vi "斯坦道溶解氧校准.vi"() -> ()   [LabVIEW 2016, in "斯坦道多参数.lvlib"]
uses:
  <vilib>/Utility/miscctls.llb/LVPointTypeDef.ctl
  <vilib>/Analysis/NI_AALBase.lvlib
  <vilib>/Analysis/NI_AALPro.lvlib
panel:
  in  "读取":bool
  out "滤波设定":dbl
  out "第二点信号值":dbl
  out "第一点信号值":dbl
  out "通讯状态":string
  in  "盐度自动获取":bool
  in  "大气压补偿":dbl format="%#.2f"
  in  "盐度补偿":dbl format="%#.2f"
  out "DO %":dbl caption="饱和度值" format="%#.2f"
  out "第二点校准值":dbl
  out "第一点校准值":dbl
  out "最小值":sgl format="%.2g"
  out "最大值":sgl format="%.2g"
  in  "校准停止":bool
  in  "校准模式":u16(ring) items=["两点校准", "单点校准"]
  in  "标液2":dbl
  in  "标液1":dbl
  out "波形图表":dbl(graph) caption="历史曲线"
  out "温度测量值":dbl caption="温度" format="%#.2f"
  out "变异系数":dbl format="%.6g"
  out "standard deviation":dbl caption="标准差" format="%0.2f"
  out "mean":dbl caption="均值" format="%0.2f"
  out "提示":string
  in  "校准启动":bool
  out "DO mg/L":dbl caption="测试值" format="%#.2f"
  out "电极斜率":dbl format="%#.6f"
  out "电极零点":dbl format="%#.6f"
  # "溶解氧电极设定"
  # "℃"
  # "%"
  # "mg/L"
  # "kPa"
  # "请选择校准模式:"
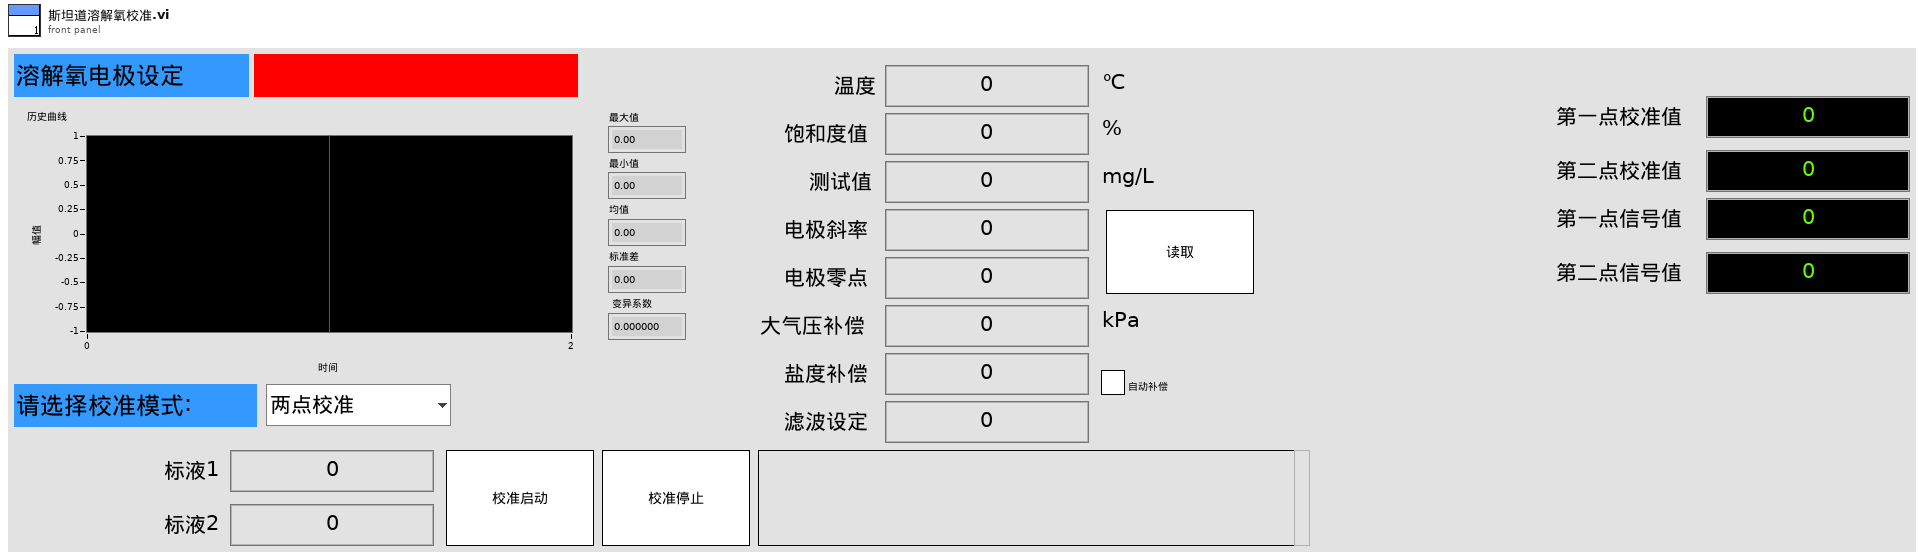
[diagram p1: front panel]
types:
  T1 = typedef "斯坦道多参数.lvlib/通知队列类型.ctl" = enum16{"pH", "DO", "DO2", "Cond", "Turb", "ORP", "叶绿素a", "藻密度", "COD"}
  T2 = typedef "LVPointTypeDef.ctl" = cluster{"Horizontal":i16, "Vertical":i16}
  T3 = cluster{"pH":u32, "DO":u32, "Cond":u32, "Turb":u32, "叶绿素a":u32, "藻密度":u32, "ORP":u32, "COD":u32}
  T4 = enum8{"Enabled", "Disabled", "Disabled and Grayed Out"}
  T5 = cluster{"ph":bool, "DO":bool, "Cond":bool, "Turb":bool, "叶绿素a":bool, "藻密度":bool, "ORP":bool, "COD":bool, "DO2":bool}
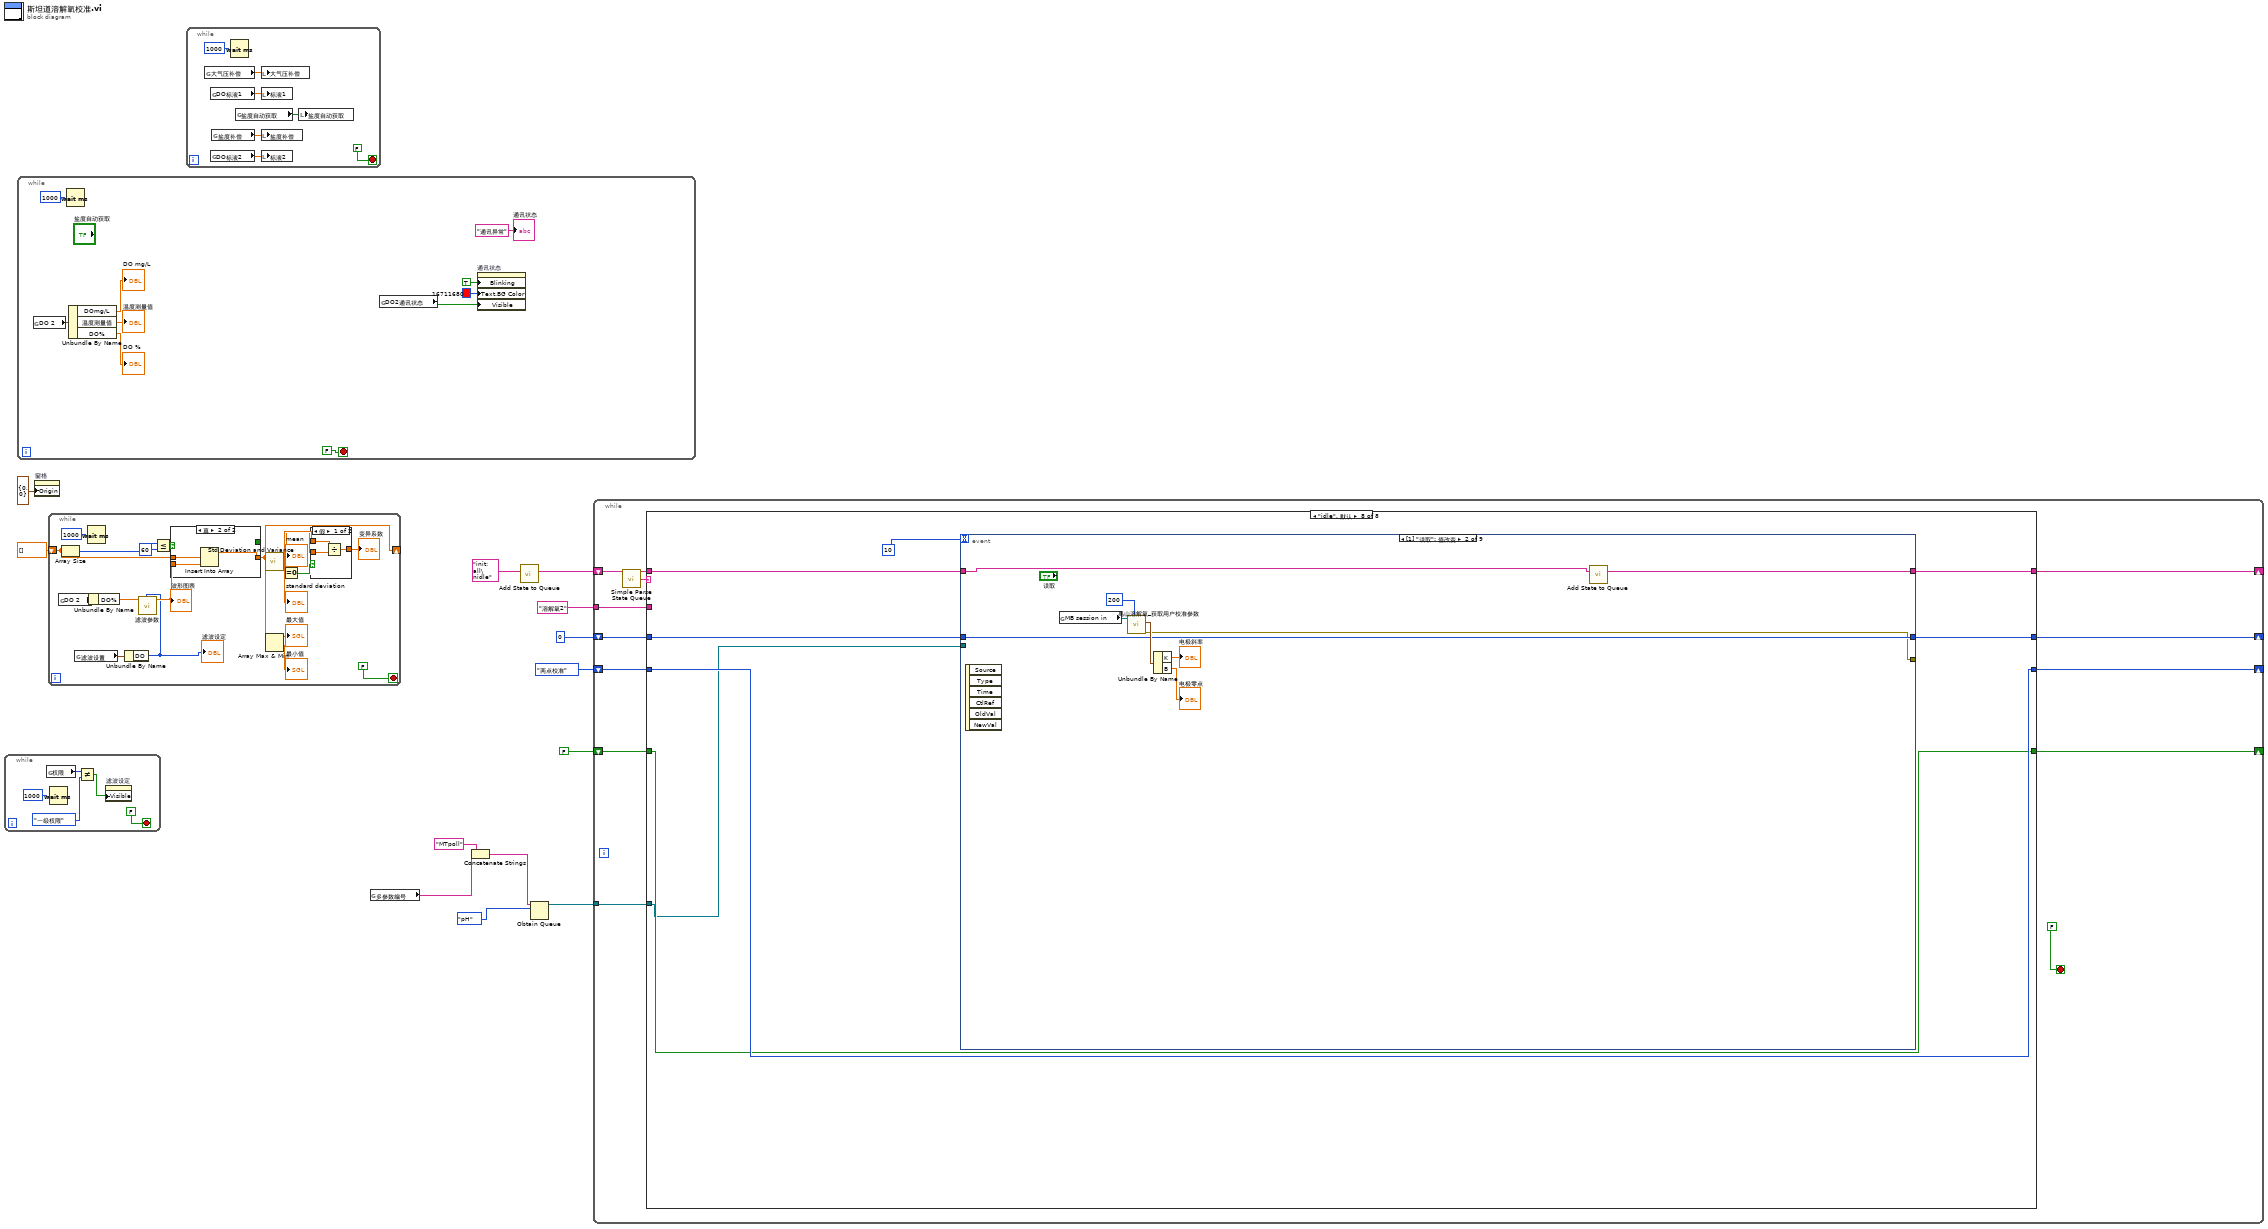
[diagram p0: block diagram]
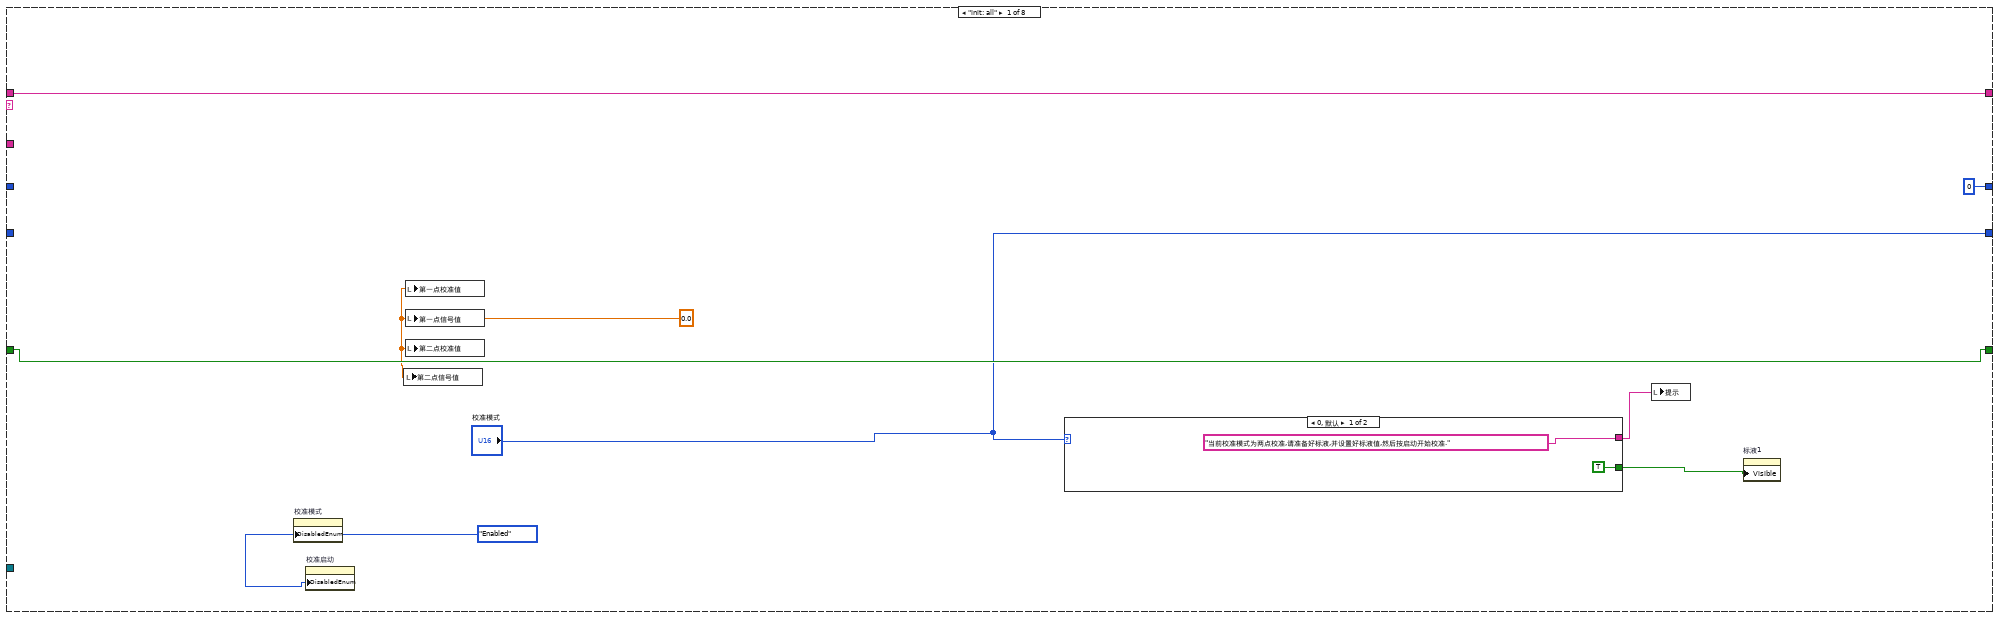
[diagram p2: hidden frame]
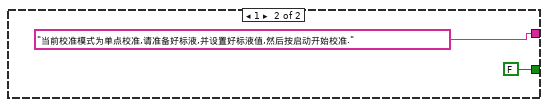
[diagram p3: hidden frame]
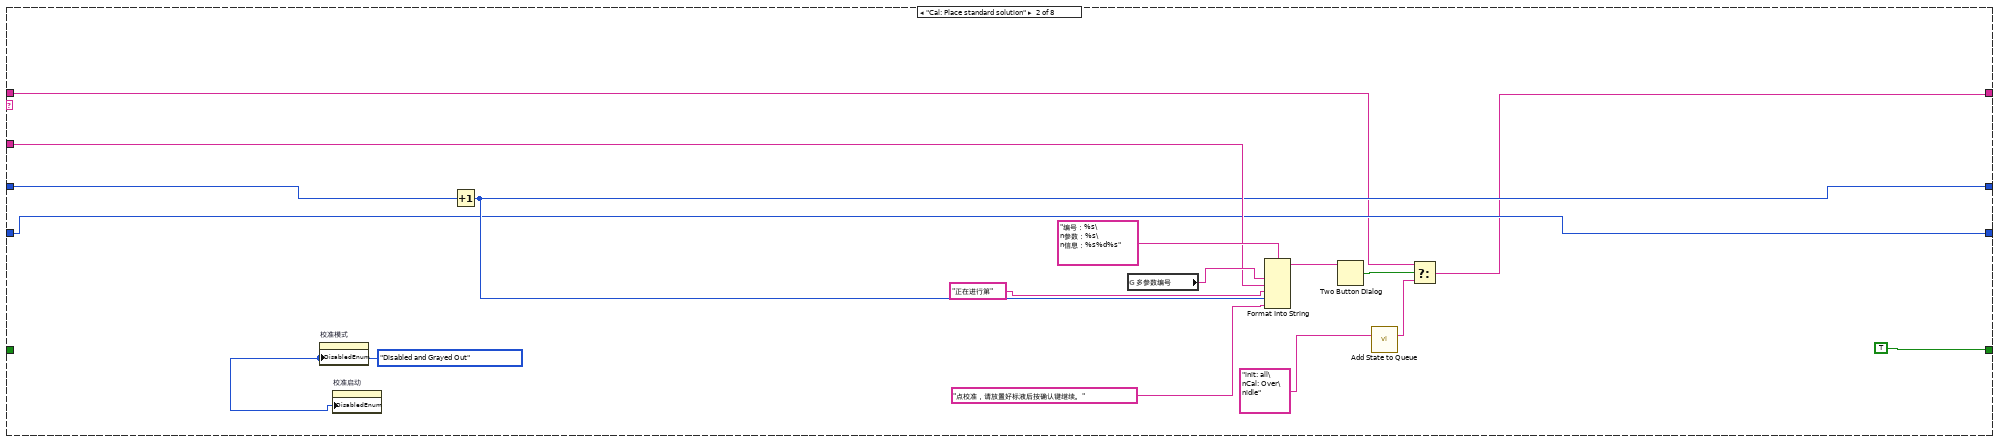
[diagram p4: hidden frame]
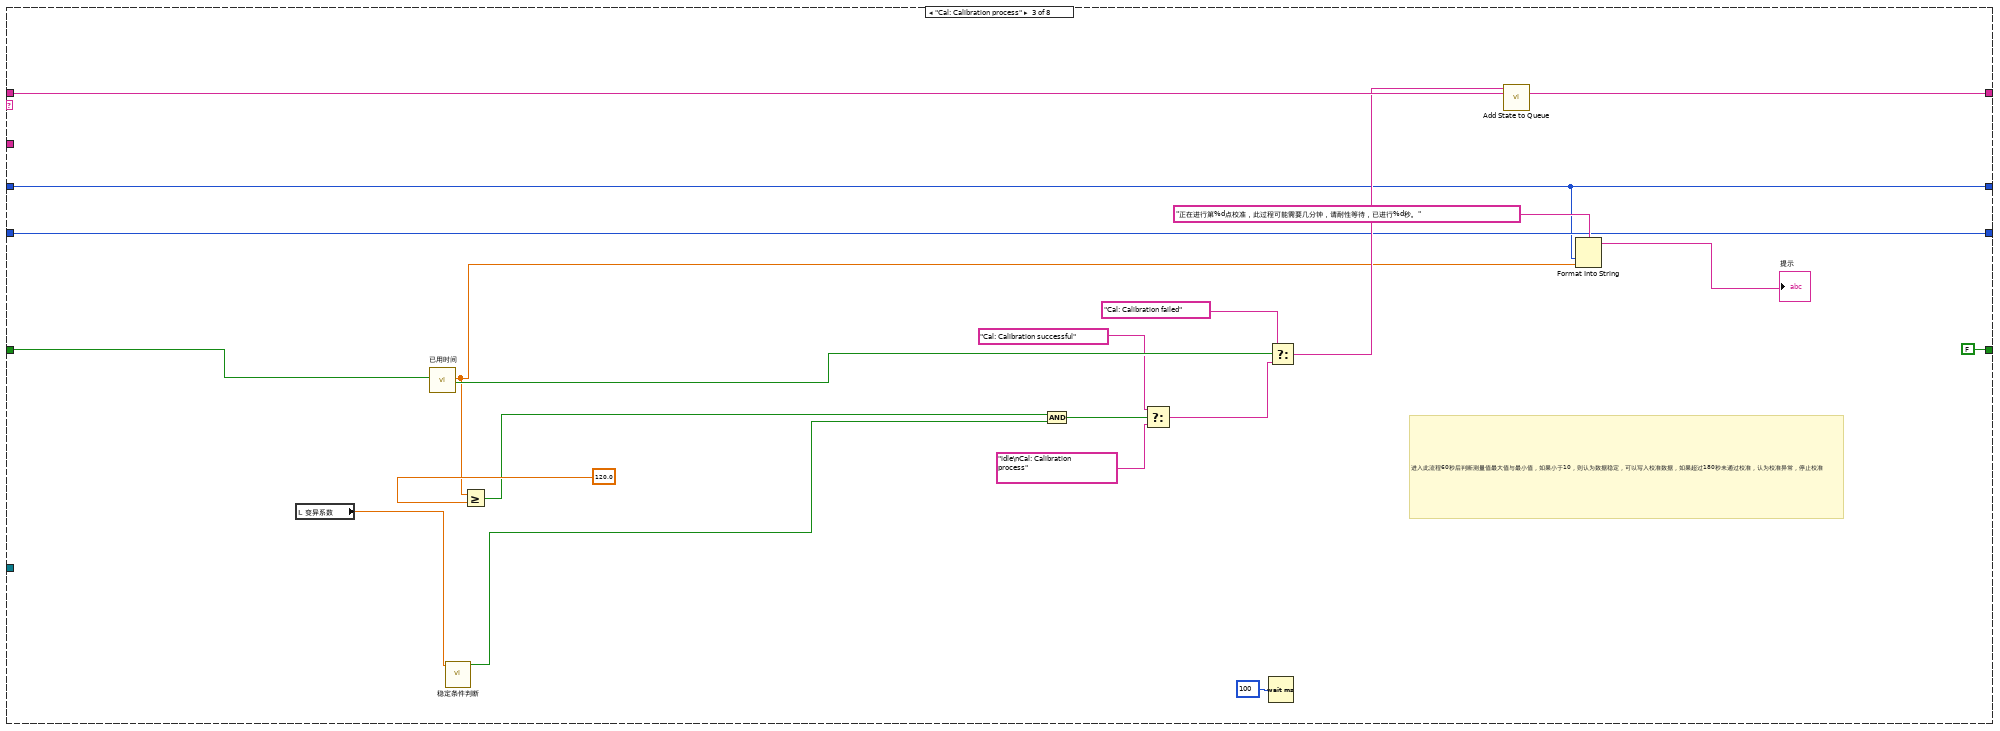
[diagram p5: hidden frame]
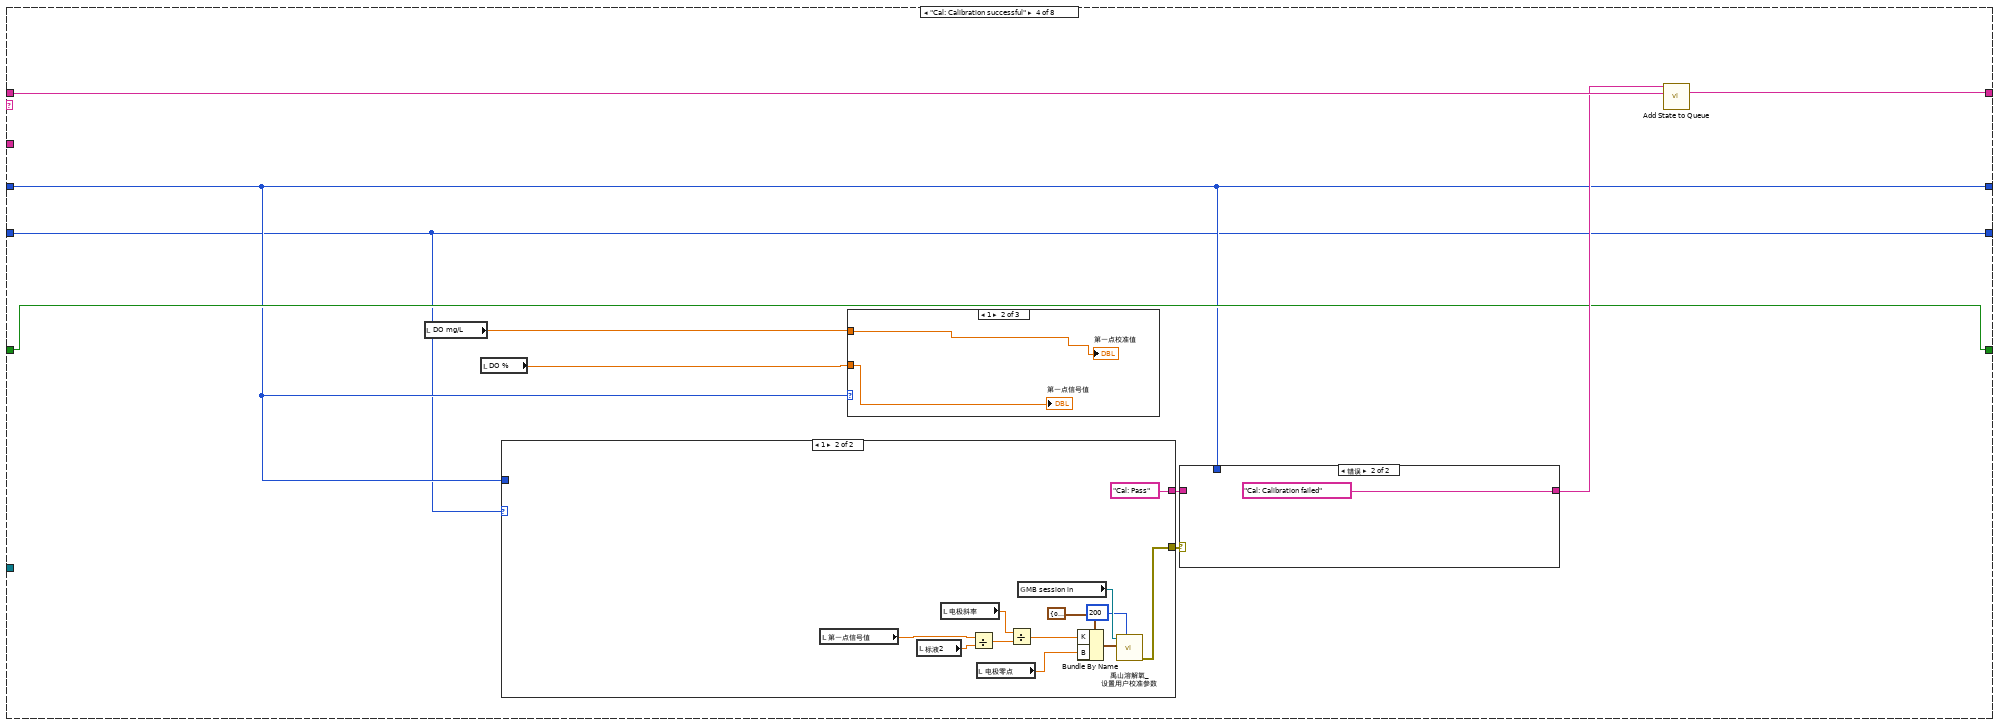
[diagram p6: hidden frame]
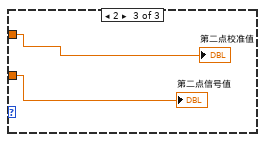
[diagram p8: hidden frame]
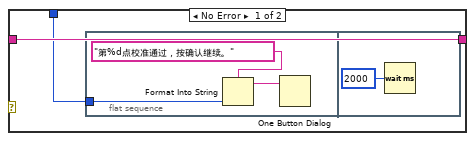
[diagram p9: hidden frame]
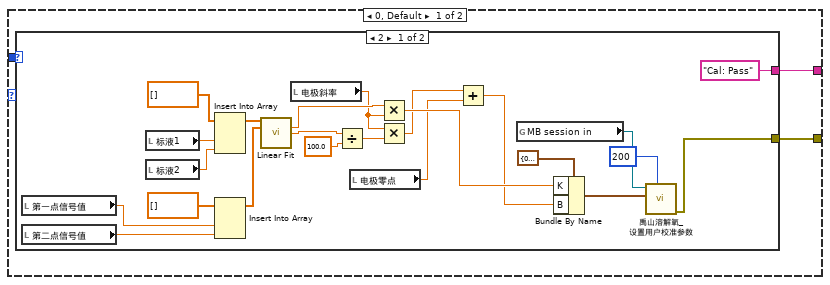
[diagram p10: hidden frame]
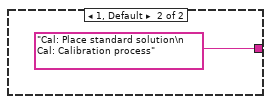
[diagram p11: hidden frame]
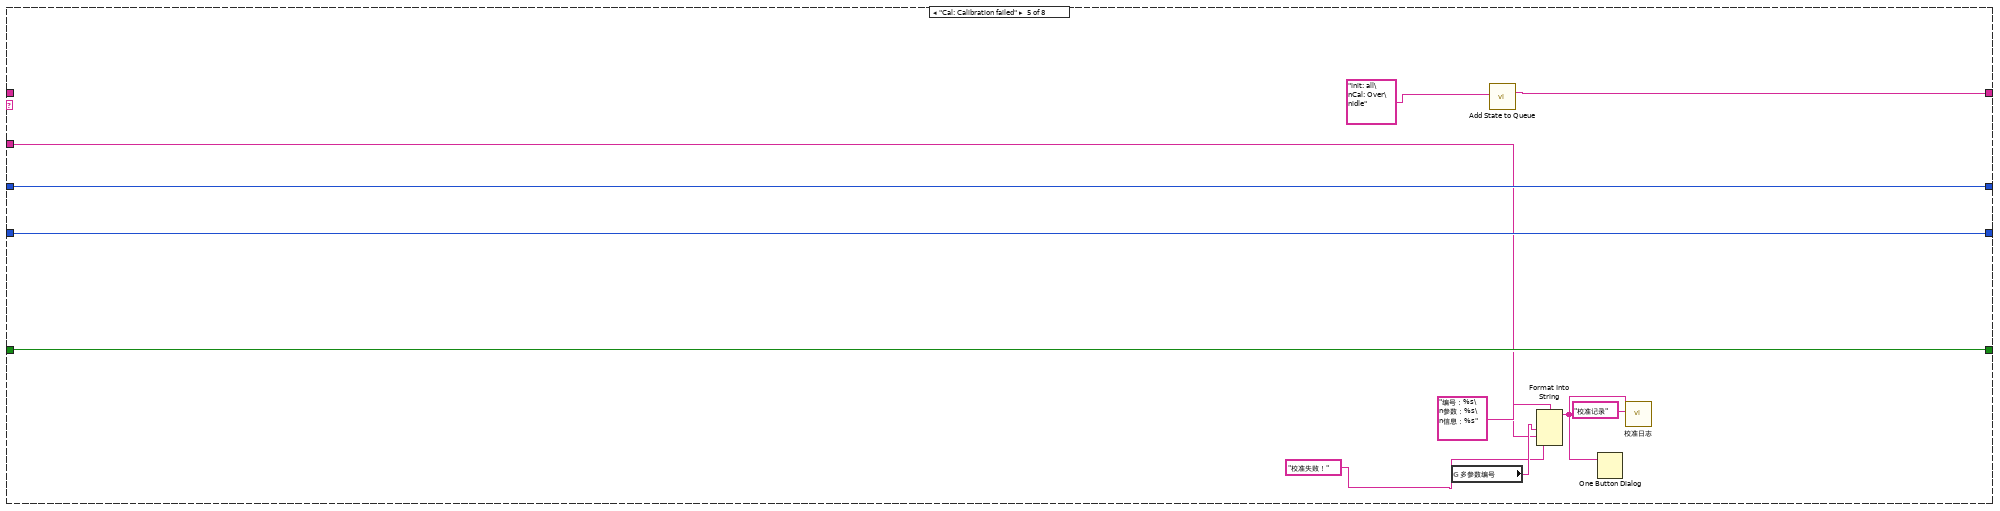
[diagram p12: hidden frame]
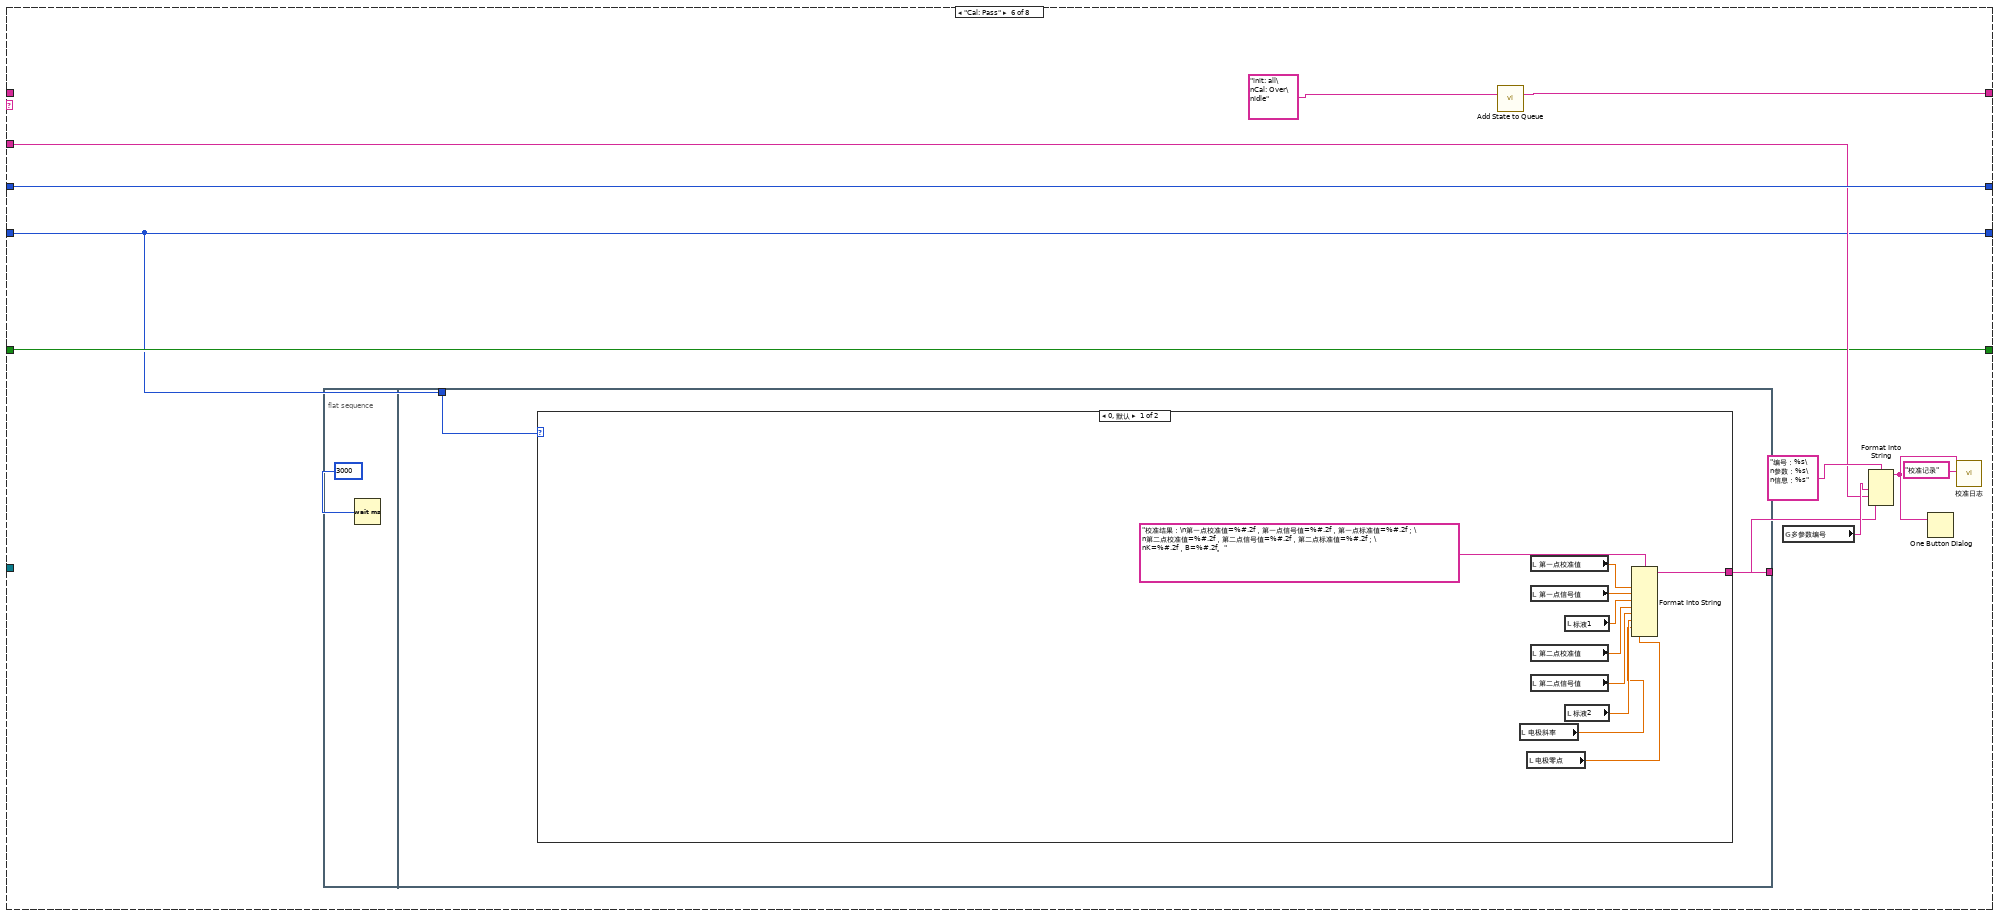
[diagram p13: hidden frame]
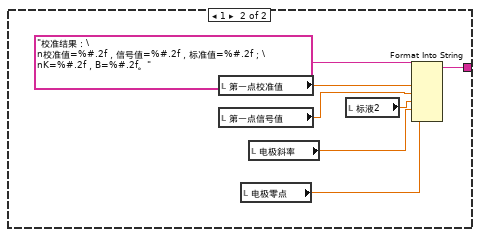
[diagram p14: hidden frame]
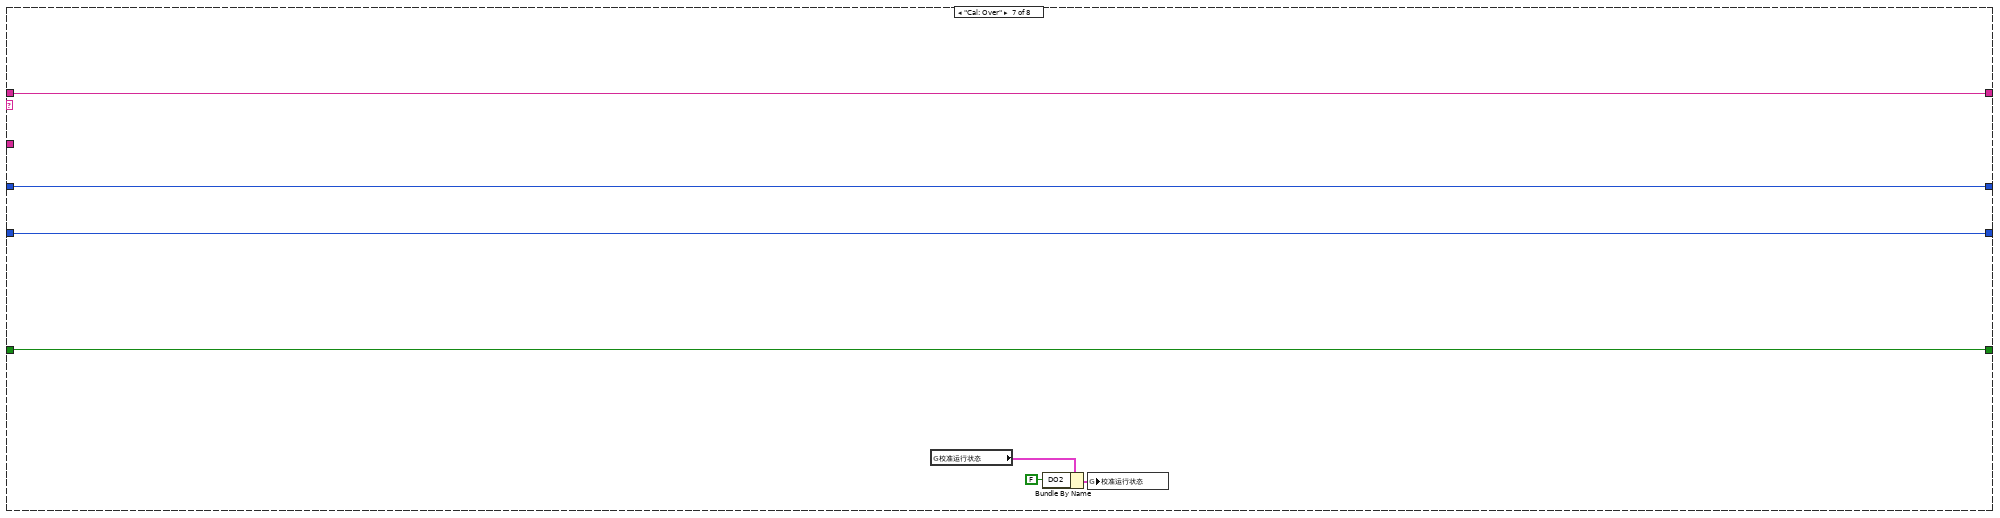
[diagram p15: hidden frame]
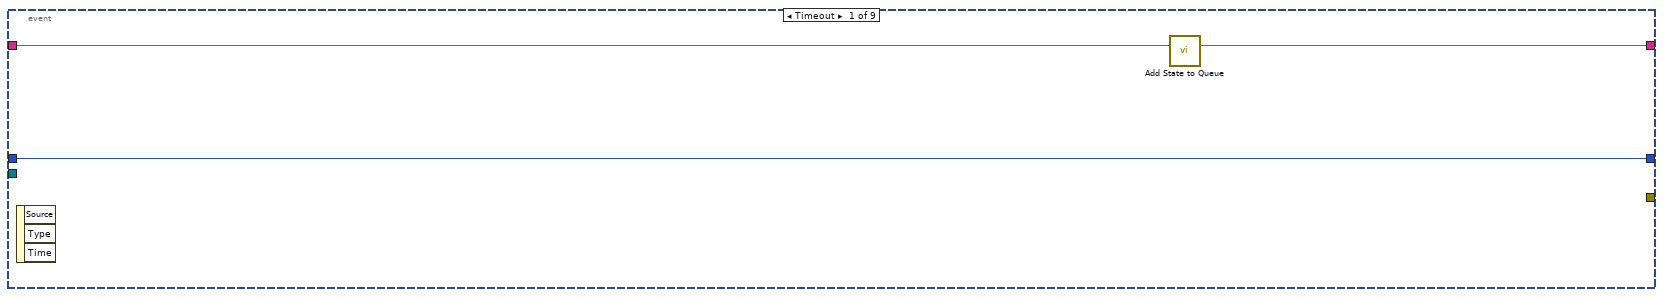
[diagram p16: hidden frame]
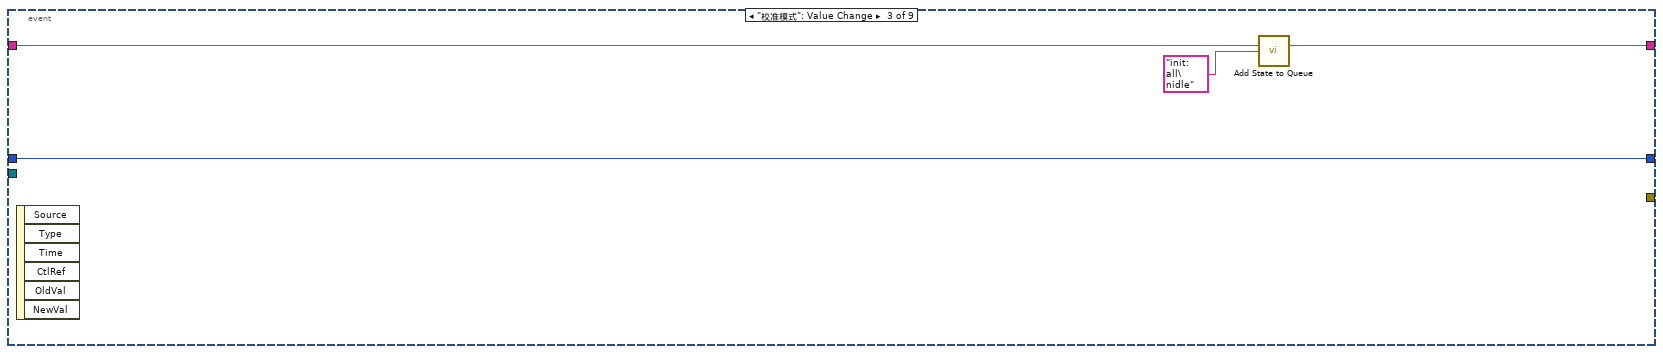
[diagram p17: hidden frame]
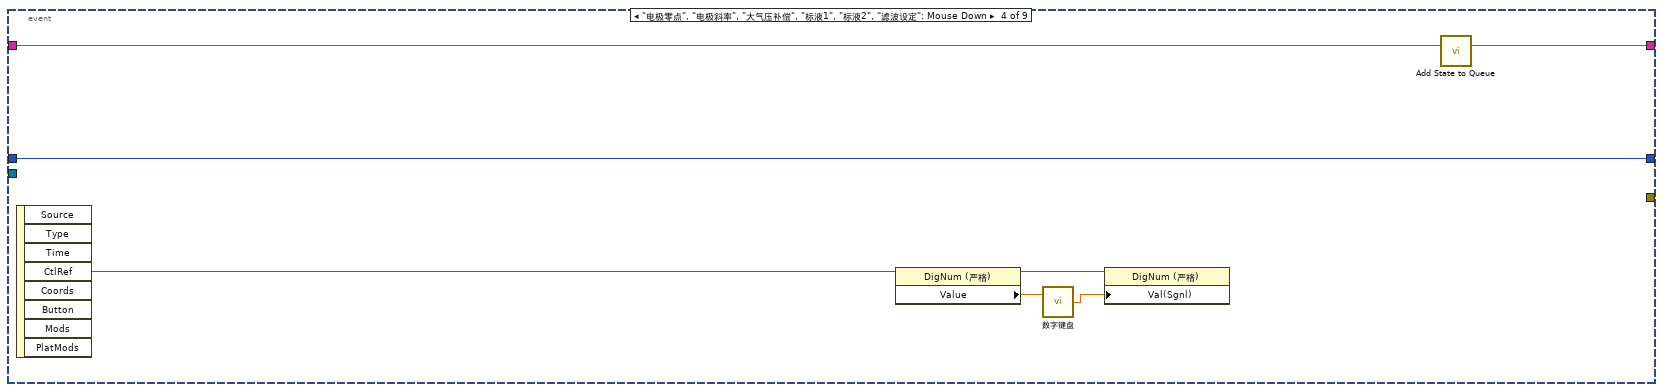
[diagram p18: hidden frame]
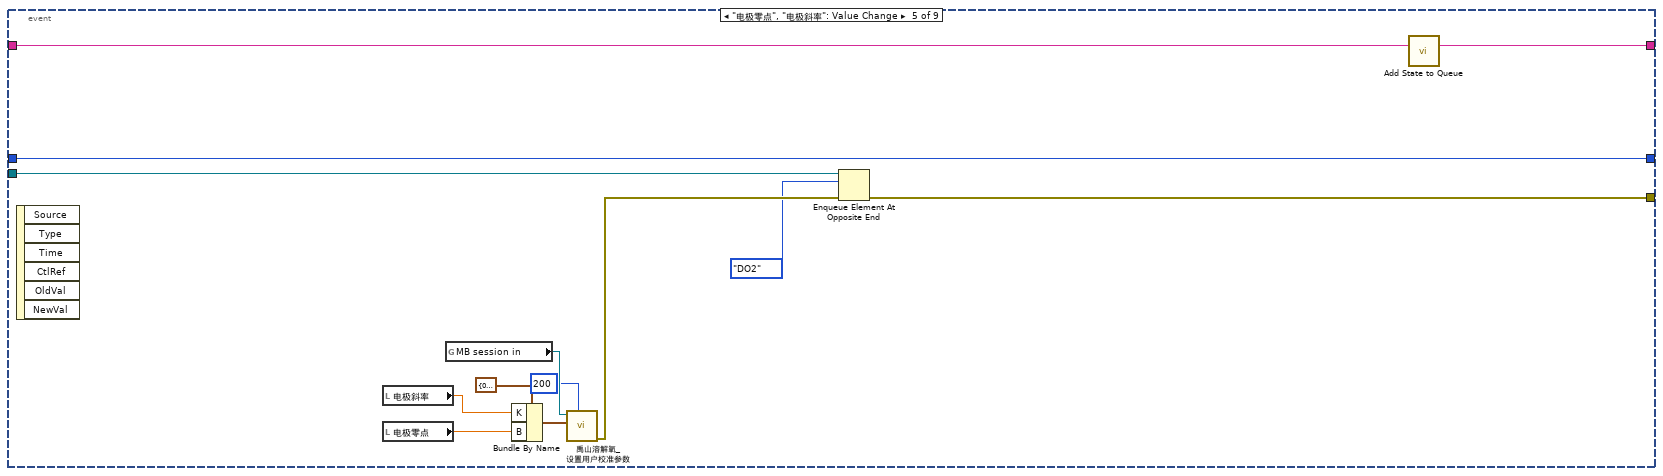
[diagram p19: hidden frame]
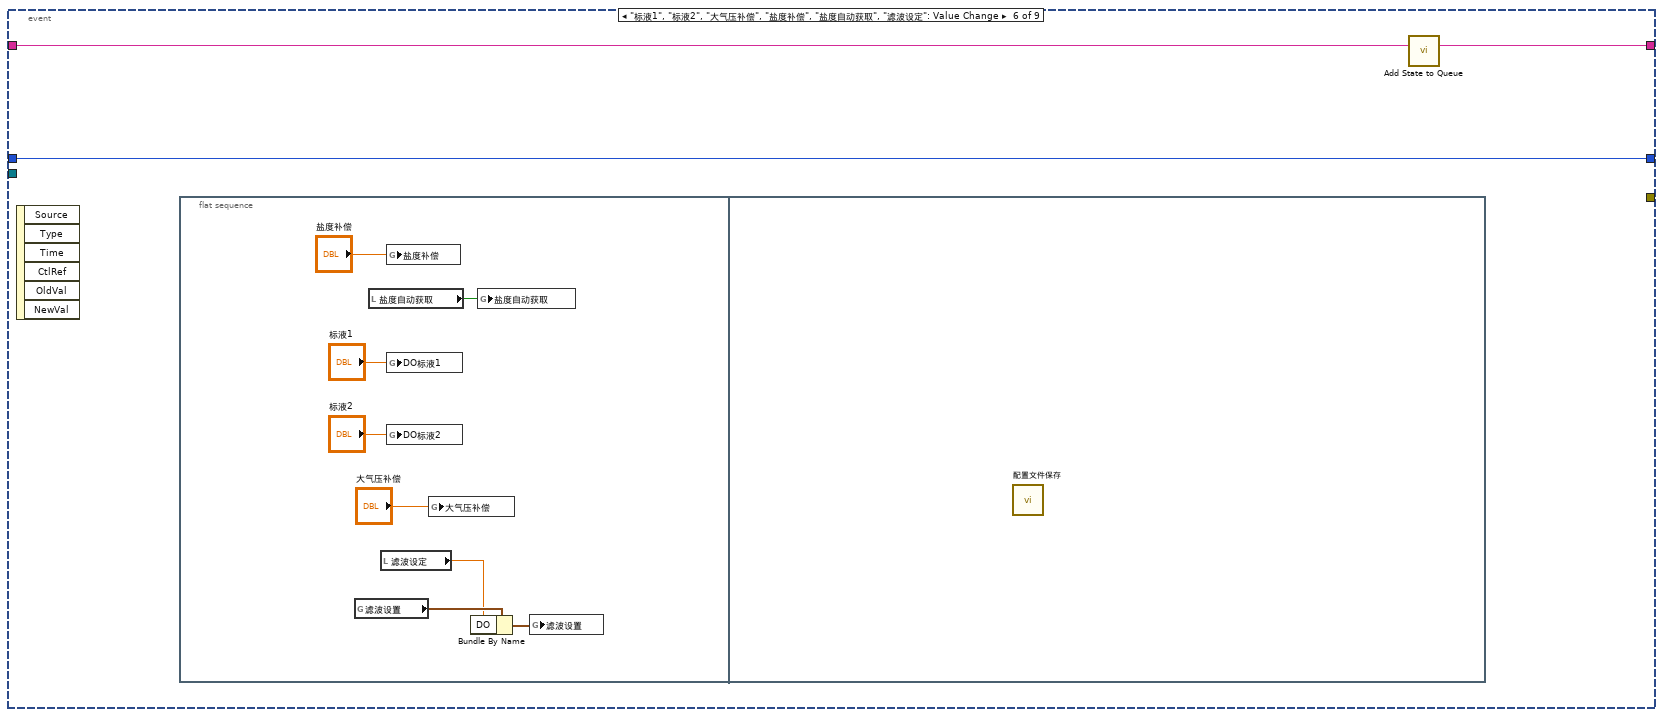
[diagram p20: hidden frame]
diagram:
  n1 = while {
    stop <- FALSE stop-if-true
    n2 = global read "多参数全局变量.vi" "权限"() -> (w17:enum16{"一级权限", "二级权限", "三级权限"})
    n3 = Wait (ms)(milliseconds to wait=u32 1000 ("等待时间（毫秒）")) -> ()  [unwired: 1 out]
    n4 = Not Equal?(x=w17, y=enum16{"一级权限", "二级权限", "三级权限"}."一级权限") -> (x != y?=w14:bool)
    n5 = property on="滤波设定" class="DigNum (严格)"("Visible"=w14) -> ()  [unwired: 2 in, 2 out]
  }
  n6 = while {
    stop <- FALSE stop-if-true
    n7 = global read "禹山过程全局变量.vi" "DO 2"() -> (w24:cluster{"温度测量值":sgl, "DO%":sgl, "DOmg/L":sgl})
    n8 = Wait (ms)(milliseconds to wait=u32 1000 ("等待时间（毫秒）")) -> ()  [unwired: 1 out]
    n9 = Unbundle By Name(w24) -> ("DOmg/L"=→"DO mg/L":sgl, "温度测量值"=→"温度测量值":sgl, "DO%"=→"DO %":sgl)
    n10 = global read "多参数全局变量.vi" "DO2通讯状态"() -> (w19:bool)
    n11 = property on="通讯状态" class="Str"("Blinking"=TRUE ("闪烁"), "Text.BG Color"=u32 16711680, "Visible"=w19) -> ()  [unwired: 2 in, 2 out]
    "通讯状态" <- "通讯异常" ("当前串口")
  }
  n12 = property on="窗格" class="Pane"("Origin"=T2 {"Horizontal"=0, "Vertical"=0} ("原点")) -> ()  [unwired: 2 in, 2 out]
  n13 = while {
    shift-right: [w35] -> _
    shift-left: sgl[] [] -> [w42]
    stop <- FALSE stop-if-true
    n14 = global read "禹山过程全局变量.vi" "DO 2"() -> (w36:cluster{"温度测量值":sgl, "DO%":sgl, "DOmg/L":sgl})
    n15 = Array Size(array=w42) -> (size(s)=w44:i32)
    n16 = global read "断电保存变量.vi" "滤波设置"() -> (w30:T3)
    n17 = Wait (ms)(milliseconds to wait=u32 1000 ("等待时间（毫秒）")) -> ()  [unwired: 1 out]
    n18 = Unbundle By Name(w36) -> ("DO%"=w32:sgl)
    n19 = Unbundle By Name(w30) -> ("DO"=w29:u32)
    "滤波设定" <- w29
    n20 = call "滤波参数.vi"("滤波次数"=w29, "x"=w32) -> ("mode"=w31:dbl)  [unwired: 9 in]
    "波形图表" <- w31
    n21 = Less Or Equal?(x=w44, y=60) -> (x <= y?=w43:bool)
    n22 = case shown="真" w43 {
      tunnel: w42 -> [w55 w58]
      tunnel: w31 -> [w53 w57]
      tunnel: [w51 w56] -> w35
      tunnel: [TRUE _] -> _
      frame False {
        n23 = Replace Array Subset(array=w55, new element=w53) -> (w54:sgl[])  [unwired: 1 in]
        n24 = Rotate 1D Array(1:w54, 2:-1 ("n")) -> (0:w51:sgl[])
      }
      frame True {
        n25 = Insert Into Array(array=w58, new element=w57) -> (w56:sgl[])  [unwired: 1 in]
      }
    }
    n26 = call <vilib>:"Std Deviation and Variance.vi"("X"=w35) -> ("mean"=w37:dbl, "standard deviation"=w38:dbl)  [unwired: 1 in, 1 out]
    "standard deviation" <- w38
    "mean" <- w37
    n27 = Array Max & Min(array=w35) -> (max value=→"最大值":sgl, min value=→"最小值":sgl)  [unwired: 2 out]
    n28 = Equal To 0?(x=w37) -> (x = 0?=w41:bool)
    n29 = case shown="假" w41 {
      tunnel: w38 -> [w49 _]
      tunnel: [w48 _] -> w40
      tunnel: w37 -> [w47 _]
      frame False {
        n30 = Divide(x=w49, y=w47) -> (x/y=w48:dbl)
      }
      frame True {
      }
    }
    "变异系数" <- w40
  }
  n31 = while {
    stop <- FALSE stop-if-true
    n32 = global read "断电保存变量.vi" "大气压补偿"() -> (w61:dbl)
    n33 = global read "断电保存变量.vi" "DO标液1"() -> (w63:dbl)
    n34 = global read "断电保存变量.vi" "DO标液2"() -> (w62:dbl)
    n35 = global read "断电保存变量.vi" "盐度补偿"() -> (w59:dbl)
    n36 = Wait (ms)(milliseconds to wait=u32 1000 ("等待时间（毫秒）")) -> ()  [unwired: 1 out]
    n37 = global read "断电保存变量.vi" "盐度自动获取"() -> (w60:bool)
    n38 = local write "大气压补偿"(w61) -> ()
    n39 = local write "标液1"(w63) -> ()
    n40 = local write "盐度补偿"(w59) -> ()
    n41 = local write "标液2"(w62) -> ()
    n42 = local write "盐度自动获取"(w60) -> ()
  }
  n43 = global read "多参数全局变量.vi" "多参数编号"() -> (w3:string)
  n44 = Concatenate Strings("MTpoll" ("名称（未命名）"), w3) -> (w4:string)
  n45 = call "Add State to Queue.vi"("State(s) In (\"\")"="init: all\nidle" ("State(s) In (\"\")")) -> ("States Out"=w10:string)  [unwired: 14 in]
  n46 = Obtain Queue(name (unnamed)=w4, element data type=通知队列类型."pH" ("枚举")) -> (queue out=w2:refnum<queue>)  [unwired: 3 in, 2 out]
  n47 = while {
    shift-right: [w74] -> _
    shift-left: w10 -> [w78]
    shift-right: [w71] -> _
    shift-left: 0 -> [w73]
    tunnel: "溶解氧2" ("State(s) In (\"\")") -> [w72]
    shift-right: [w69] -> _
    shift-left: enum16{"两点校准", "单点校准"}."两点校准" ("校准模式") -> [w70]
    shift-right: [w67] -> _
    shift-left: FALSE -> [w68]
    tunnel: w2 -> [w66]
    stop <- FALSE stop-if-true
    n48 = call "Simple Parse State Queue.vi"("State Queue"=w78) -> ("Remain States"=w75:string, "Next State"=w76:string)  [unwired: 13 in]
    n49 = case shown="\"idle\", 默认" w76 {
      tunnel: w75 -> [w86 w94 w126 w135 _ _ w236 w244]
      tunnel: [w86 w93 w125 w134 w195 w200 w236 w243] -> w74
      tunnel: w73 -> [_ w102 w111 w129 w198 w209 w235 w241]
      tunnel: w72 -> [_ w103 _ _ w189 w205 _ _]
      tunnel: [0 w100 w111 w129 w198 w209 w235 w242] -> w71
      tunnel: w70 -> [_ w99 w112 w128 w197 w201 w234 w240]
      tunnel: ["校准模式" w99 w112 w128 w197 w201 w234 w240] -> w69
      tunnel: w68 -> [w83 _ w114 w130 w196 w204 w233 w238]
      tunnel: [w83 TRUE FALSE w130 w196 w204 w233 w238] -> w67
      tunnel: w66 -> [_ _ _ _ _ _ _ w237]
      frame "init: all" {
        w81 = T4."Enabled" ("禁用")
        w82 = 0.0 ("第一点校准值")
        n50 = property on="校准模式" class="Ring (严格)"("DisabledEnum"=w81) -> ()  [unwired: 2 in, 2 out]
        n51 = property on="校准启动" class="Bool"("DisabledEnum"=w81) -> ()  [unwired: 2 in, 2 out]
        n52 = local write "第二点信号值"(w82) -> ()
        n53 = local write "第一点校准值"(w82) -> ()
        n54 = local write "第一点信号值"(w82) -> ()
        n55 = local write "第二点校准值"(w82) -> ()
        n56 = case shown="0, 默认" "校准模式" {
          tunnel: ["当前校准模式为两点校准,请准备好标液,并设置好标液值,然后按启动开始校准." ("提示") "当前校准模式为单点校准,请准备好标液,并设置好标液值,然后按启动开始校准." ("提示")] -> w85
          tunnel: [TRUE ("可见") FALSE ("可见")] -> w79
          frame 0, Default {
          }
          frame 1 {
          }
        }
        n57 = local write "提示"(w85) -> ()
        n58 = property on="标液1" class="DigNum (严格)"("Visible"=w79) -> ()  [unwired: 2 in, 2 out]
      }
      frame "Cal: Place standard solution" {
        w92 = T4."Disabled and Grayed Out" ("禁用")
        n59 = property on="校准模式" class="Ring (严格)"("DisabledEnum"=w92) -> ()  [unwired: 2 in, 2 out]
        n60 = property on="校准启动" class="Bool"("DisabledEnum"=w92) -> ()  [unwired: 2 in, 2 out]
        n61 = Increment(x=w102) -> (x+1=w100:i32)
        n62 = global read "多参数全局变量.vi" "多参数编号"() -> (w105:string)
        n63 = Format Into String(format string="编号：%s\n参数：%s\n信息：%s%d%s" ("格式字符串"), w105, w103, "正在进行第" ("消息"), w100, "点校准，请放置好标液后按确认键继续。" ("消息")) -> (resulting string=w97:string)  [unwired: 2 in, 1 out]
        n64 = Two Button Dialog(message=w97) -> (T button?=w96:bool)  [unwired: 2 in]
        n65 = call "Add State to Queue.vi"("State(s) In (\"\")"="init: all\nCal: Over\nidle" ("State(s) In (\"\")")) -> ("States Out"=w95:string)  [unwired: 14 in]
        n66 = Select(t=w94, s=w96, f=w95) -> (s? t:f=w93:string)
      }
      frame "Cal: Calibration process" {
        # "进入此流程60秒后判断测量值最大值与最小值，如果小于10，则认为数据稳定，可以写入校准数据，如果超过180秒未通过校准，认为校准异常，停止校准"
        n67 = local read "变异系数"() -> (w108:dbl)
        n68 = call "已用时间"("Reset"=w114) -> ("Elapsed Time (s)"=w110:dbl, "Time has Elapsed"=w127:bool)  [unwired: 11 in, 6 out]
        n69 = call "稳定条件判断.vi"("变异系数"=w108) -> ("布尔"=w107:bool)  [unwired: 10 in]
        n70 = Greater Or Equal?(x=w110, y=120.0) -> (x >= y?=w122:bool)
        n71 = And(x=w122, y=w107) -> (x .and. y?=w119:bool)
        n72 = Select(t="Cal: Calibration successful" ("State(s) In (\"\")"), s=w119, f="idle\nCal: Calibration process" ("State(s) In (\"\")")) -> (s? t:f=w118:string)
        n73 = Wait (ms)(milliseconds to wait=u32 100 ("等待时间（毫秒）")) -> ()  [unwired: 1 out]
        n74 = Select(t="Cal: Calibration failed" ("State(s) In (\"\")"), s=w127, f=w118) -> (s? t:f=w117:string)
        n75 = call "Add State to Queue.vi"("State(s) In Front (\"\")"=w117, "State(s) In (\"\")"=w126) -> ("States Out"=w125:string)  [unwired: 13 in]
        n76 = Format Into String(format string="正在进行第%d点校准，此过程可能需要几分钟，请耐性等待，已进行%d秒。" ("格式字符串"), w111, w110) -> (resulting string=→"提示":string)  [unwired: 2 in, 1 out]
      }
      frame "Cal: Calibration successful" {
        n77 = local read "DO mg/L"() -> (w131:dbl)
        n78 = local read "DO %"() -> (w132:dbl)
        n79 = case shown="1" w128 {
          tunnel: [w151 w177] -> w137
          tunnel: [w150 "Cal: Pass" ("State(s) In (\"\")")] -> w136
          tunnel: w129 -> [w149 _]
          frame 0, Default {
            n80 = case shown="2" w149 {
              tunnel: [w153 _] -> w151
              tunnel: ["Cal: Pass" ("State(s) In (\"\")") "Cal: Place standard solution\n Cal: Calibration process" ("State(s) In (\"\")")] -> w150
              frame 2 {
                n81 = local read "第一点信号值"() -> (w172:dbl)
                n82 = local read "第二点信号值"() -> (w171:dbl)
                n83 = local read "标液1"() -> (w169:dbl)
                n84 = local read "标液2"() -> (w168:dbl)
                n85 = Insert Into Array(array=dbl[] [] ("Weight"), new element #1=w169, new element #2=w168) -> (w167:dbl[])  [unwired: 1 in]
                n86 = Insert Into Array(array=dbl[] [] ("Weight"), new element #1=w172, new element #2=w171) -> (w166:dbl[])  [unwired: 1 in]
                n87 = call <vilib>:"Linear Fit.vi"("Y"=w167, "X"=w166) -> ("slope"=w162:dbl, "intercept"=w159:dbl)  [unwired: 9 in, 3 out]
                n88 = local read "电极斜率"() -> (w160:dbl)
                n89 = Divide(x=w159, y=100.0) -> (x/y=w155:dbl)
                n90 = local read "电极零点"() -> (w157:dbl)
                n91 = Multiply(x=w162, y=w160) -> (x*y=w161:dbl)
                n92 = Multiply(x=w160, y=w155) -> (x*y=w158:dbl)
                n93 = Add(x=w158, y=w157) -> (x+y=w156:dbl)
                n94 = global read "多参数全局变量.vi" "MB session in"() -> (w165:refnum<class "MB_Master.lvclass">)
                n95 = Bundle By Name(cluster=cluster{"K":sgl, "B":sgl} {"K"=0.0, "B"=0.0} ("用户校准参数"), "K"=w161, "B"=w156) -> (w164:cluster{"K":sgl, "B":sgl})
                n96 = call "禹山溶解氧_设置用户校准参数.vi"("Slave ID"=u8 200, "用户校准参数"=w164, "MB session in"=w165) -> ("error out"=w153:errorcluster)  [unwired: 7 in, 1 out]
              }
              frame 1, Default {
              }
            }
          }
          frame 1 {
            n97 = local read "第一点信号值"() -> (w182:dbl)
            n98 = local read "标液2"() -> (w181:dbl)
            n99 = local read "电极斜率"() -> (w179:dbl)
            n100 = Divide(x=w182, y=w181) -> (x/y=w178:dbl)
            n101 = local read "电极零点"() -> (w183:dbl)
            n102 = Divide(x=w179, y=w178) -> (x/y=w180:dbl)
            n103 = global read "多参数全局变量.vi" "MB session in"() -> (w186:refnum<class "MB_Master.lvclass">)
            n104 = Bundle By Name(cluster=cluster{"K":sgl, "B":sgl} {"K"=0.0, "B"=0.0} ("用户校准参数"), "K"=w180, "B"=w183) -> (w185:cluster{"K":sgl, "B":sgl})
            n105 = call "禹山溶解氧_设置用户校准参数.vi"("Slave ID"=u8 200, "用户校准参数"=w185, "MB session in"=w186) -> ("error out"=w177:errorcluster)  [unwired: 7 in, 1 out]
          }
        }
        n106 = case shown="1" w129 {
          tunnel: w132 -> [_ w139 w141]
          tunnel: w131 -> [_ w138 w140]
          frame 0, Default {
          }
          frame 1 {
            "第一点信号值" <- w139
            "第一点校准值" <- w138
          }
          frame 2 {
            "第二点信号值" <- w141
            "第二点校准值" <- w140
          }
        }
        n107 = case shown="错误" w137 {
          tunnel: w136 -> [w143 _]
          tunnel: [w143 "Cal: Calibration failed" ("State(s) In (\"\")")] -> w133
          tunnel: w129 -> [w142 _]
          frame No Error {
            n108 = flat-sequence {
              tunnel: w142 -> [w144]
              frame #0 {
                n109 = Format Into String(format string="第%d点校准通过，按确认继续。" ("格式字符串"), w144) -> (resulting string=w146:string)  [unwired: 2 in, 1 out]
                n110 = One Button Dialog(message=w146) -> ()  [unwired: 1 in, 1 out]
              }
              frame #1 {
                n111 = Wait (ms)(milliseconds to wait=u32 2000 ("等待时间（毫秒）")) -> ()  [unwired: 1 out]
              }
            }
          }
          frame Error {
          }
        }
        n112 = call "Add State to Queue.vi"("State(s) In Front (\"\")"=w133, "State(s) In (\"\")"=w135) -> ("States Out"=w134:string)  [unwired: 13 in]
      }
      frame "Cal: Calibration failed" {
        n113 = global read "多参数全局变量.vi" "多参数编号"() -> (w192:string)
        n114 = call "Add State to Queue.vi"("State(s) In (\"\")"="init: all\nCal: Over\nidle" ("State(s) In (\"\")")) -> ("States Out"=w195:string)  [unwired: 14 in]
        n115 = Format Into String(format string="编号：%s\n参数：%s\n信息：%s" ("格式字符串"), w192, w189, "校准失败！" ("消息")) -> (resulting string=w191:string)  [unwired: 2 in, 1 out]
        n116 = One Button Dialog(message=w191) -> ()  [unwired: 1 in, 1 out]
        n117 = call "校准日志.vi"("table"="校准记录", "日志信息"=w191) -> ()  [unwired: 9 in, 1 out]
      }
      frame "Cal: Pass" {
        n118 = flat-sequence {
          tunnel: [w212] -> w202
          tunnel: w201 -> [w211]
          frame #0 {
            n119 = Wait (ms)(milliseconds to wait=u32 3000 ("等待时间（毫秒）")) -> ()  [unwired: 1 out]
          }
          frame #1 {
            n120 = case shown="0, 默认" w211 {
              tunnel: [w222 w229] -> w212
              frame 0, Default {
                n121 = local read "电极斜率"() -> (w214:dbl)
                n122 = local read "电极零点"() -> (w213:dbl)
                n123 = local read "第一点校准值"() -> (w220:dbl)
                n124 = local read "第一点信号值"() -> (w221:dbl)
                n125 = local read "第二点校准值"() -> (w217:dbl)
                n126 = local read "第二点信号值"() -> (w216:dbl)
                n127 = local read "标液1"() -> (w218:dbl)
                n128 = local read "标液2"() -> (w215:dbl)
                n129 = Format Into String(format string="校准结果：\n第一点校准值=%#.2f，第一点信号值=%#.2f，第一点标准值=%#.2f；\n第二点校准值=%#.2f，第二点信号值=%#.2f，第二点标准值=%#.2f；\nK=%#.2f，B=%#.2f。" ("提示"), w220, w221, w218, w217, w216, w215, w214, w213) -> (resulting string=w222:string)  [unwired: 2 in, 1 out]
              }
              frame 1 {
                n130 = local read "第一点校准值"() -> (w228:dbl)
                n131 = local read "第一点信号值"() -> (w226:dbl)
                n132 = local read "电极零点"() -> (w223:dbl)
                n133 = local read "电极斜率"() -> (w224:dbl)
                n134 = local read "标液2"() -> (w225:dbl)
                n135 = Format Into String(format string="校准结果：\n校准值=%#.2f，信号值=%#.2f，标准值=%#.2f；\nK=%#.2f，B=%#.2f。" ("提示"), w228, w226, w225, w224, w223) -> (resulting string=w229:string)  [unwired: 2 in, 1 out]
              }
            }
          }
        }
        n136 = call "Add State to Queue.vi"("State(s) In (\"\")"="init: all\nCal: Over\nidle" ("State(s) In (\"\")")) -> ("States Out"=w200:string)  [unwired: 14 in]
        n137 = global read "多参数全局变量.vi" "多参数编号"() -> (w206:string)
        n138 = Format Into String(format string="编号：%s\n参数：%s\n信息：%s" ("格式字符串"), w206, w205, w202) -> (resulting string=w203:string)  [unwired: 2 in, 1 out]
        n139 = One Button Dialog(message=w203) -> ()  [unwired: 1 in, 1 out]
        n140 = call "校准日志.vi"("table"="校准记录", "日志信息"=w203) -> ()  [unwired: 9 in, 1 out]
      }
      frame "Cal: Over" {
        n141 = global read "多参数全局变量.vi" "校准运行状态"() -> (w231:T5)
        n142 = Bundle By Name(cluster=w231, "DO2"=FALSE ("DO")) -> (w232:T5)
        n143 = global write "多参数全局变量.vi" "校准运行状态"(w232) -> ()
      }
      frame "idle", Default {
        n144 = event shown="[1] \"读取\": 值改变" {
          selector: _ -> [_ _ _ _ _ _ _ _ _]
          dyn-events: _ -> [_ _ _ _ _ _ _ _ _]
          timeout: 10 -> [_ _ _ _ _ _ _ _ _]
          tunnel: [_ w250 _ _ w271 _ _ _ _] -> _
          tunnel: w244 -> [w247 w249 w260 w265 w272 w281 w292 w307 _]
          tunnel: [w246 w248 w259 w266 w279 w282 w294 w306 w309] -> w243
          tunnel: [w245 w251 w257 w267 w280 w283 w293 w304 w310] -> w242
          tunnel: w241 -> [w245 w251 w257 w267 w280 w283 w293 w304 w310]
          tunnel: w237 -> [_ _ _ _ w270 _ _ _ _]
          event Timeout {
            n145 = event-data() -> ()  [unwired: 1 in, 3 out]
            n146 = call "Add State to Queue.vi"("State(s) In (\"\")"=w247) -> ("States Out"=w246:string)  [unwired: 14 in]
          }
          event "读取": Value Change {
            n147 = event-data() -> ()  [unwired: 1 in, 6 out]
            n148 = global read "多参数全局变量.vi" "MB session in"() -> (w255:refnum<class "MB_Master.lvclass">)
            n149 = call "禹山溶解氧_获取用户校准参数.vi"("y"=u16 200, "MB session in"=w255) -> ("error out"=w250:errorcluster, "输出值"=w252:cluster{"K":sgl, "B":sgl})  [unwired: 7 in, 1 out]
            n150 = Unbundle By Name(w252) -> ("K"=→"电极斜率":sgl, "B"=→"电极零点":sgl)
            n151 = call "Add State to Queue.vi"("State(s) In (\"\")"=w249) -> ("States Out"=w248:string)  [unwired: 14 in]
          }
          event "校准模式": Value Change {
            n152 = event-data() -> ()  [unwired: 1 in, 6 out]
            n153 = call "Add State to Queue.vi"("State(s) In (\"\")"=w260, "State(s) At Back (\"\")"="init: all\nidle" ("State(s) In (\"\")")) -> ("States Out"=w259:string)  [unwired: 13 in]
          }
          event "电极零点", "电极斜率", "大气压补偿", "标液1", "标液2", "滤波设定": Mouse Down {
            n154 = event-data() -> ("CtlRef"=w264:refnum<vi>)  [unwired: 1 in, 7 out]
            n155 = property class="DigNum (严格)"(reference=w264) -> (reference out=w261:refnum<vi>, "Value"=w262:dbl)  [unwired: 1 in, 1 out]
            n156 = call "数字键盘.vi"("OldNumber"=w262) -> ("NewNumber"=w263:dbl)  [unwired: 1 in]
            n157 = property class="DigNum (严格)"(reference=w261, "Val(Sgnl)"=w263) -> ()  [unwired: 1 in, 2 out]
            n158 = call "Add State to Queue.vi"("State(s) In (\"\")"=w265) -> ("States Out"=w266:string)  [unwired: 14 in]
          }
          event "电极零点", "电极斜率": Value Change {
            n159 = event-data() -> ()  [unwired: 1 in, 6 out]
            n160 = local read "电极斜率"() -> (w276:dbl)
            n161 = local read "电极零点"() -> (w275:dbl)
            n162 = global read "多参数全局变量.vi" "MB session in"() -> (w274:refnum<class "MB_Master.lvclass">)
            n163 = Bundle By Name(cluster=cluster{"K":sgl, "B":sgl} {"K"=0.0, "B"=0.0} ("用户校准参数"), "K"=w276, "B"=w275) -> (w277:cluster{"K":sgl, "B":sgl})
            n164 = call "禹山溶解氧_设置用户校准参数.vi"("Slave ID"=u8 200, "用户校准参数"=w277, "MB session in"=w274) -> ("error out"=w273:errorcluster)  [unwired: 7 in, 1 out]
            n165 = Enqueue Element At Opposite End(queue=w270, element=通知队列类型."DO2" ("枚举"), error in (no error)=w273) -> (error out=w271:errorcluster)  [unwired: 1 in, 2 out]
            n166 = call "Add State to Queue.vi"("State(s) In (\"\")"=w272) -> ("States Out"=w279:string)  [unwired: 14 in]
          }
          event "标液1", "标液2", "大气压补偿", "盐度补偿", "盐度自动获取", "滤波设定": Value Change {
            n167 = event-data() -> ()  [unwired: 1 in, 6 out]
            n168 = flat-sequence {
              frame #0 {
                n169 = global read "断电保存变量.vi" "滤波设置"() -> (w286:T3)
                n170 = local read "盐度自动获取"() -> (w287:bool)
                n171 = local read "滤波设定"() -> (w284:dbl)
                n172 = global write "断电保存变量.vi" "盐度补偿"("盐度补偿") -> ()
                n173 = global write "断电保存变量.vi" "DO标液1"("标液1") -> ()
                n174 = global write "断电保存变量.vi" "DO标液2"("标液2") -> ()
                n175 = global write "断电保存变量.vi" "大气压补偿"("大气压补偿") -> ()
                n176 = Bundle By Name(cluster=w286, "DO"=w284) -> (w285:T3)
                n177 = global write "断电保存变量.vi" "盐度自动获取"(w287) -> ()
                n178 = global write "断电保存变量.vi" "滤波设置"(w285) -> ()
              }
              frame #1 {
                n179 = call "配置文件保存.vi"() -> ()  [unwired: 12 in]
              }
            }
            n180 = call "Add State to Queue.vi"("State(s) In (\"\")"=w281) -> ("States Out"=w282:string)  [unwired: 14 in]
          }
          event "盐度补偿": Mouse Down {
            n181 = event-data() -> ("CtlRef"=w295:refnum<vi>)  [unwired: 1 in, 7 out]
            n182 = local read "盐度自动获取"() -> (w296:bool)
            n183 = case shown="假" w296 {
              tunnel: w295 -> [w297 _]
              frame False {
                n184 = property class="DigNum (严格)"(reference=w297) -> (reference out=w298:refnum<vi>, "Value"=w299:dbl)  [unwired: 1 in, 1 out]
                n185 = call "数字键盘.vi"("OldNumber"=w299) -> ("NewNumber"=w300:dbl)  [unwired: 1 in]
                n186 = property class="DigNum (严格)"(reference=w298, "Val(Sgnl)"=w300) -> ()  [unwired: 1 in, 2 out]
              }
              frame True {
              }
            }
            n187 = call "Add State to Queue.vi"("State(s) In (\"\")"=w292) -> ("States Out"=w294:string)  [unwired: 14 in]
          }
          event "校准启动": Value Change {
            n188 = event-data() -> ()  [unwired: 1 in, 6 out]
            n189 = global read "多参数全局变量.vi" "校准运行状态"() -> (w302:T5)
            n190 = Bundle By Name(cluster=w302, "DO2"=TRUE ("DO")) -> (w303:T5)
            n191 = call "Add State to Queue.vi"("State(s) In (\"\")"=w307, "State(s) At Back (\"\")"="init: all\nCal: Place standard solution\n Cal: Calibration process\nidle" ("State(s) In (\"\")")) -> ("States Out"=w306:string)  [unwired: 13 in]
            n192 = global write "多参数全局变量.vi" "校准运行状态"(w303) -> ()
          }
          event "校准停止": Value Change {
            n193 = event-data() -> ()  [unwired: 1 in, 6 out]
            n194 = call "Add State to Queue.vi"("State(s) In (\"\")"="init: all\nCal: Over\nidle" ("State(s) In (\"\")")) -> ("States Out"=w309:string)  [unwired: 14 in]
          }
        }
      }
    }
  }
